vi "addNormalDistributedNoise.vi"(0 "Array":dbl[](array[numeric]), 1 "mean":dbl, 2 "initialize":bool=TRUE, 3 "seed":i32=-1, 4 "standard deviation":dbl=1.0 format="%0.2f") -> (5 "added Noise Array":dbl[](array[numeric]))   [LabVIEW 2021]
uses:
  <vilib>/Analysis/NI_AALBase.lvlib
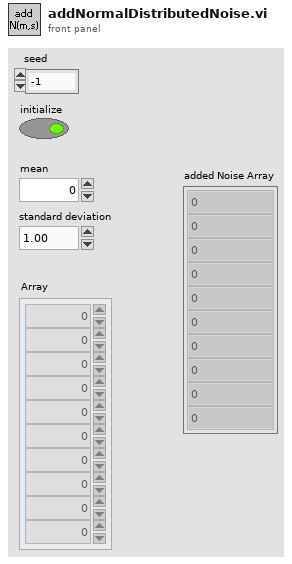
[diagram p1: front panel]
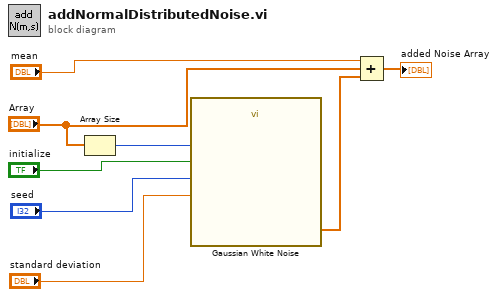
[diagram p0: block diagram]
diagram:
  n1 = Array Size(array="Array") -> (size(s)=w8:i32)
  n2 = call <vilib>:"Gaussian White Noise.vi"("initialize?"="initialize", "seed"="seed", "standard deviation"="standard deviation", "samples"=w8) -> ("Gaussian noise pattern"=w5:dbl[])  [unwired: 6 in, 1 out]
  n3 = Compound Arithmetic op=ADD("mean", "Array", w5) -> (→"added Noise Array":dbl[])
